vi "min_jerk_trajectory_start_target_start.vi"(0 "Initial Position":dbl, 5 "Start Position":dbl=1.0, 7 "Target Position":dbl=1.0, 9 "Initial Time [s]":dbl, 11 "Time For 1 Transition [s]":dbl=1.0, 12 "Pause duration at target [s]":dbl=1.0, 13 "Delta Time [s]":dbl=0.001) -> (8 "Profile":cluster{"time (s)":dbl, "setpoint":dbl}[](array[cluster]) {"setpoint" format="%.2f"; "time (s)" format="%.3f"})   [LabVIEW 2019]
panel:
  out "XY Graph":cluster{"X":dbl, "Y":dbl}[](graph)
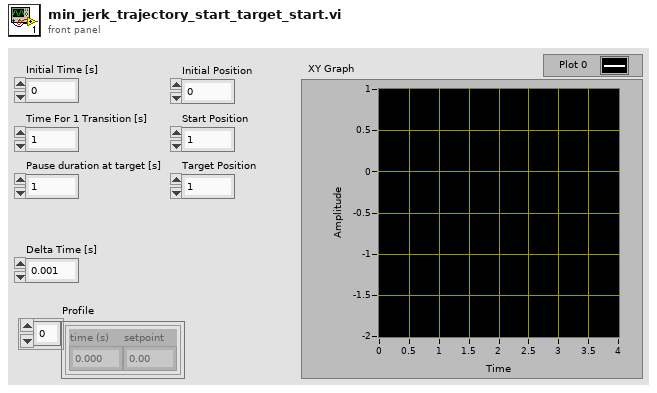
[diagram p1: front panel]
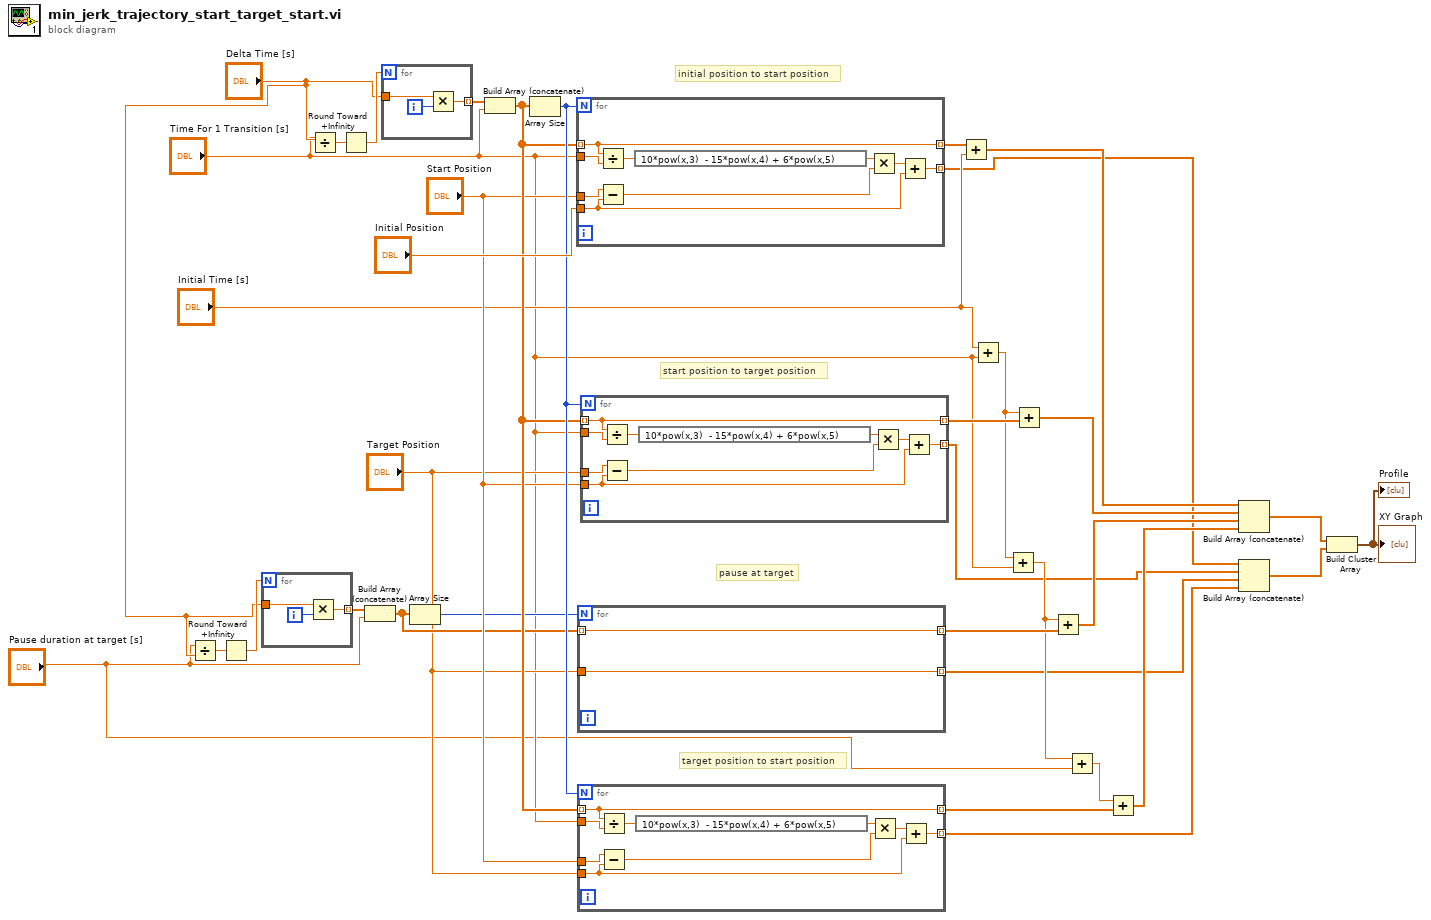
[diagram p0: block diagram]
diagram:
  # "target position to start position"
  # "pause at target"
  # "start position to target position"
  # "initial position to start position"
  n1 = Divide(x="Pause duration at target [s]", y="Delta Time [s]") -> (x/y=w22:dbl)
  n2 = Round Toward +Infinity(x=w22) -> (ceil(x): smallest int >= x=w23:dbl)
  n3 = for {
    N: w23 -> [_]
    tunnel: "Delta Time [s]" -> [w37]
    tunnel: [w36] -> w24 mode=indexing
    i -> [w38]
    n4 = Multiply(x=w37, y=w38) -> (x*y=w36:dbl)
  }
  n5 = Divide(x="Time For 1 Transition [s]", y="Delta Time [s]") -> (x/y=w34:dbl)
  n6 = Round Toward +Infinity(x=w34) -> (ceil(x): smallest int >= x=w33:dbl)
  n7 = Build Array (concatenate)(w24, "Pause duration at target [s]") -> (w19:dbl[])
  n8 = for {
    N: w33 -> [_]
    tunnel: "Delta Time [s]" -> [w40]
    tunnel: [w39] -> w32 mode=indexing
    i -> [w41]
    n9 = Multiply(x=w40, y=w41) -> (x*y=w39:dbl)
  }
  n10 = Array Size(array=w19) -> (size(s)=w20:i32)
  n11 = Build Array (concatenate)(w32, "Time For 1 Transition [s]") -> (w28:dbl[])
  n12 = Array Size(array=w28) -> (size(s)=w29:i32)
  n13 = for {
    N: w29 -> [_]
    tunnel: [w47] -> w4 mode=indexing
    tunnel: [w43] -> w30 mode=indexing
    tunnel: "Time For 1 Transition [s]" -> [w46]
    tunnel: w28 -> [w43] mode=indexing
    tunnel: "Start Position" -> [w45]
    tunnel: "Initial Position" -> [w44]
    n14 = Divide(x=w43, y=w46) -> (x/y=w42:dbl)
    n15 = Subtract(x=w45, y=w44) -> (x-y=w48:dbl)
    n16 = expression code="10*pow(x,3)  - 15*pow(x,4) + 6*pow(x,5)"(w42) -> (w49:dbl)
    n17 = Multiply(x=w49, y=w48) -> (x*y=w50:dbl)
    n18 = Add(x=w50, y=w44) -> (x+y=w47:dbl)
  }
  n19 = for {
    N: w20 -> [_]
    tunnel: [w52] -> w15 mode=indexing
    tunnel: w19 -> [w52] mode=indexing
    tunnel: [w51] -> w5 mode=indexing
    tunnel: "Target Position" -> [w51]
  }
  n20 = for {
    N: w29 -> [_]
    tunnel: [w58] -> w6 mode=indexing
    tunnel: [w54] -> w11 mode=indexing
    tunnel: "Time For 1 Transition [s]" -> [w57]
    tunnel: w28 -> [w54] mode=indexing
    tunnel: "Start Position" -> [w56]
    tunnel: "Target Position" -> [w55]
    n21 = Divide(x=w54, y=w57) -> (x/y=w53:dbl)
    n22 = Subtract(x=w56, y=w55) -> (x-y=w59:dbl)
    n23 = expression code="10*pow(x,3)  - 15*pow(x,4) + 6*pow(x,5)"(w53) -> (w60:dbl)
    n24 = Multiply(x=w60, y=w59) -> (x*y=w61:dbl)
    n25 = Add(x=w61, y=w55) -> (x+y=w58:dbl)
  }
  n26 = for {
    N: w29 -> [_]
    tunnel: [w67] -> w3 mode=indexing
    tunnel: [w63] -> w25 mode=indexing
    tunnel: "Time For 1 Transition [s]" -> [w66]
    tunnel: w28 -> [w63] mode=indexing
    tunnel: "Target Position" -> [w65]
    tunnel: "Start Position" -> [w64]
    n27 = Divide(x=w63, y=w66) -> (x/y=w62:dbl)
    n28 = Subtract(x=w65, y=w64) -> (x-y=w68:dbl)
    n29 = expression code="10*pow(x,3)  - 15*pow(x,4) + 6*pow(x,5)"(w62) -> (w69:dbl)
    n30 = Multiply(x=w69, y=w68) -> (x*y=w70:dbl)
    n31 = Add(x=w70, y=w64) -> (x+y=w67:dbl)
  }
  n32 = Add(x=w30, y="Initial Time [s]") -> (x+y=w7:dbl[])
  n33 = Add(x="Initial Time [s]", y="Time For 1 Transition [s]") -> (x+y=w17:dbl)
  n34 = Add(x=w17, y="Time For 1 Transition [s]") -> (x+y=w14:dbl)
  n35 = Add(x=w17, y=w25) -> (x+y=w8:dbl[])
  n36 = Add(x=w14, y=w15) -> (x+y=w9:dbl[])
  n37 = Add(x=w14, y="Pause duration at target [s]") -> (x+y=w12:dbl)
  n38 = Add(x=w12, y=w11) -> (x+y=w10:dbl[])
  n39 = Build Array (concatenate)(w7, w8, w9, w10) -> (w2:dbl[])
  n40 = Build Array (concatenate)(w4, w3, w5, w6) -> (w1:dbl[])
  n41 = Build Cluster Array(w2, w1) -> (→"Profile" →"XY Graph":cluster{dbl, "Target Position":dbl}[])
